vi "Close Last FITS Reference.vi"(8 "error in (no error)":errorcluster, 11 "Save Image in":refnum<class "Save Image.lvclass">) -> (0 "error out":errorcluster, 3 "Save Image out":refnum<class "Save Image.lvclass">)   [LabVIEW 2018, in "Save Image.lvclass"]
uses:
  Save Image.lvclass
  <userlib>/gfitsio/gfitsio.lvlib
  Simulated_Header/Simulated_Header.lvclass
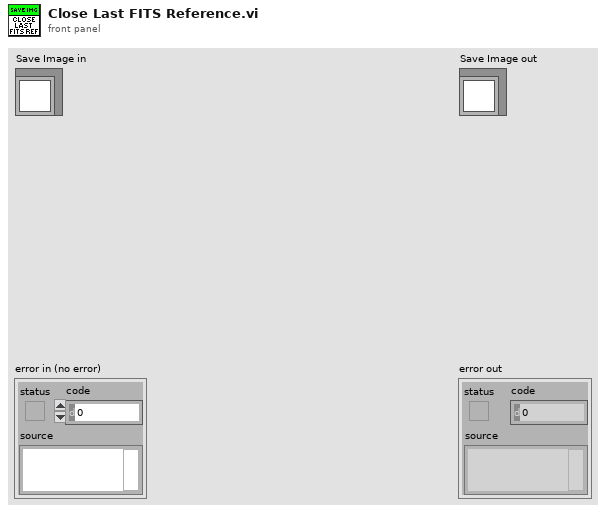
[diagram p1: front panel]
types:
  T1 = typedef "gfitsio.lvlib/gfitsio-refnum.ctl" = refnum<k1>
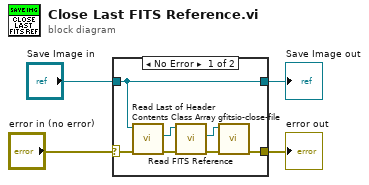
[diagram p0: block diagram]
diagram:
  n1 = case shown="No Error" "error in (no error)" {
    selector: "error in (no error)" -> [w9 w13]
    tunnel: [w11 w13] -> w3
    tunnel: [w10 w12] -> w1
    tunnel: "Save Image in" -> [w10 w12]
    frame No Error {
      n2 = call "Read Last of Header Contents Class Array.vi"("error in (no error)"=w9, "Save Image in"=w10) -> ("error out"=w7:errorcluster, "Simulated_Header.lvclass"=w8:refnum<class "Simulated_Header.lvclass">)  [unwired: 7 in, 1 out]
      n3 = call "Read FITS Reference.vi"("error in (no error)"=w7, "Simulated_Header in"=w8) -> ("error out"=w6:errorcluster, "gfits refnum"=w5:T1)  [unwired: 7 in, 1 out]
      n4 = call <userlib>:"gfitsio-close-file.vi"("error in (no error)"=w6, "gfits refnum"=w5) -> ("error out"=w11:errorcluster)  [unwired: 8 in, 1 out]
    }
    frame Error {
    }
  }
  "error out" <- w3
  "Save Image out" <- w1
